vi "Target location.vi"(11 "Display map":dbl[][](array[numeric])) -> (2 "target location":dbl[](array[numeric]))   [LabVIEW 2015]
panel:
  in  "Priority map":dbl[][](array[numeric])
  in  "robot location":dbl[](array[numeric])
  out "distances":dbl[](array[numeric])
  out "Indices":i32[][](array[numeric])
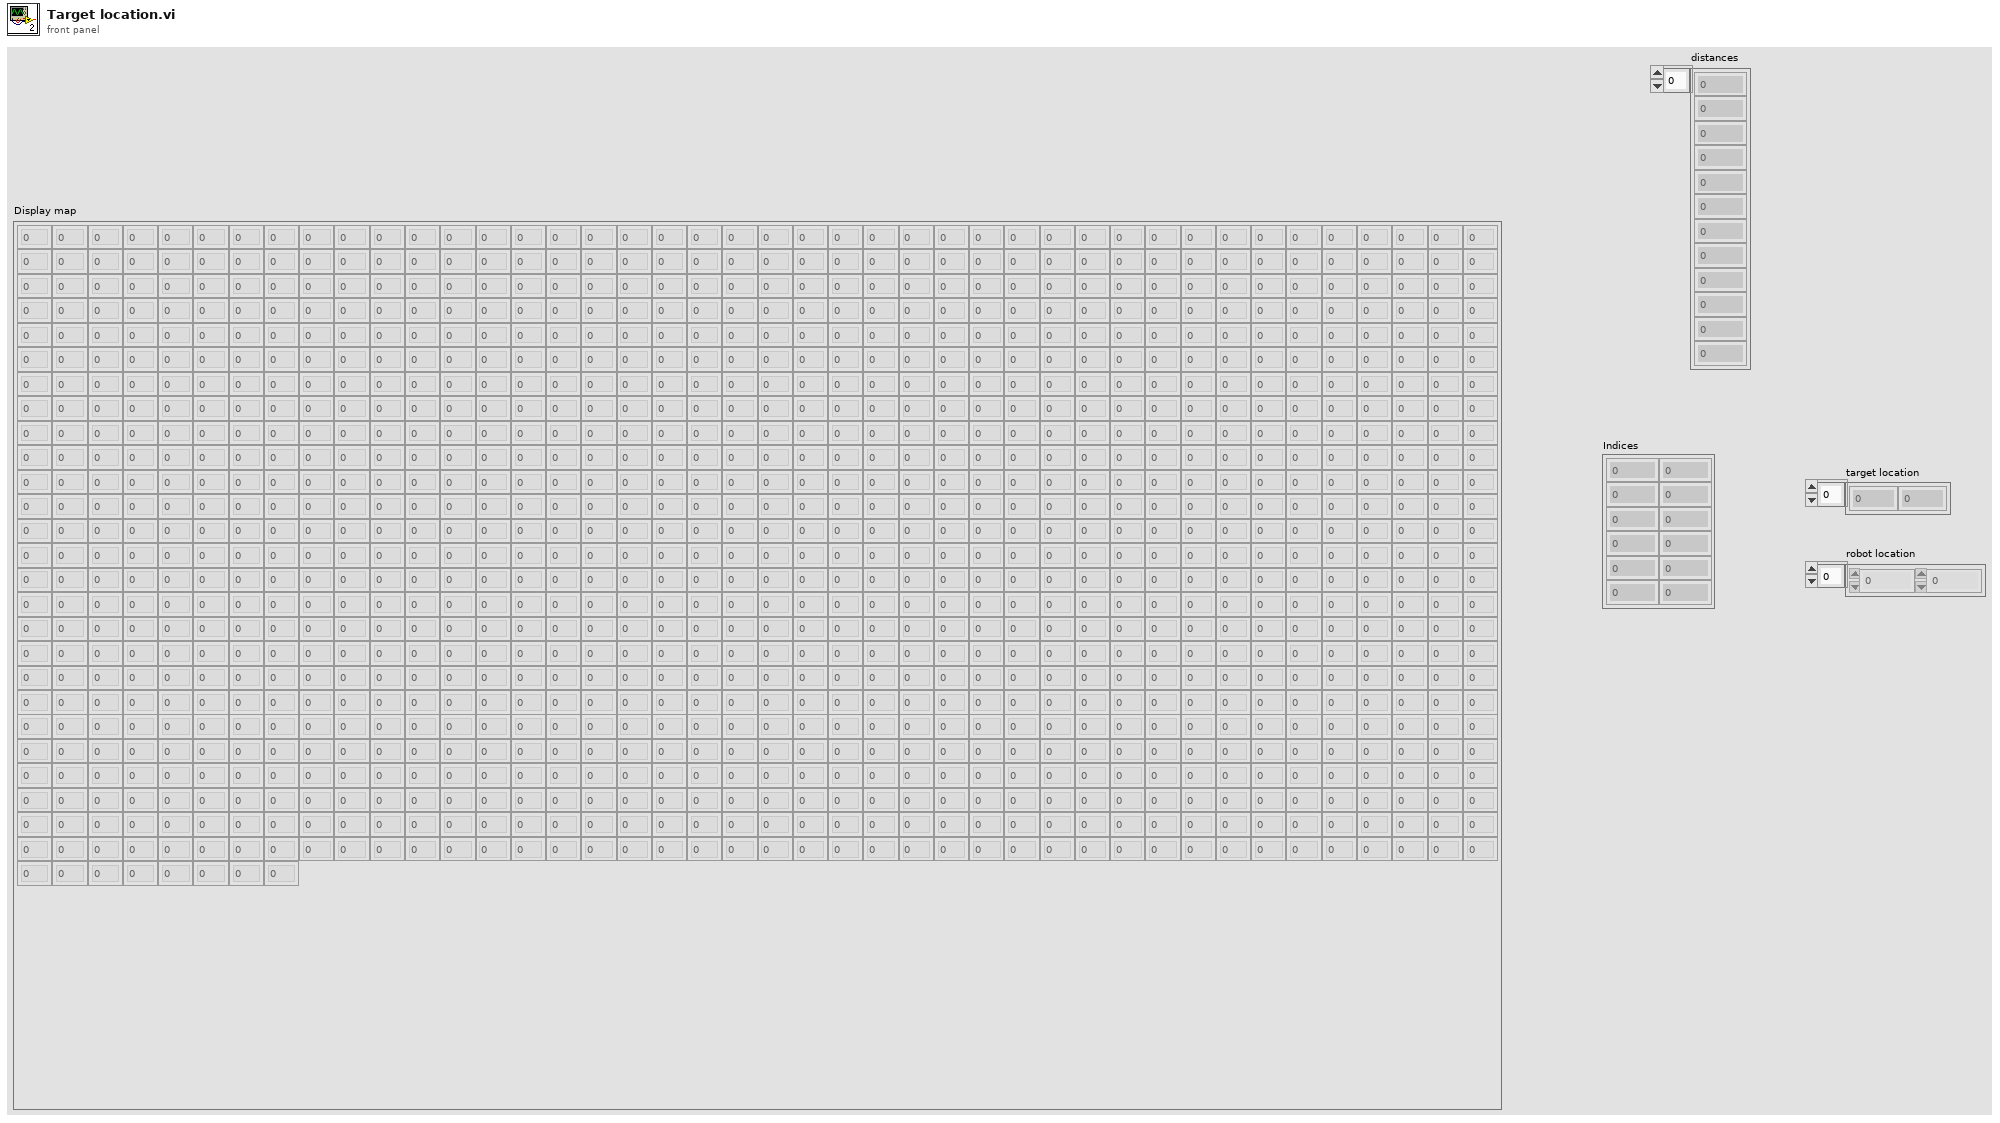
[diagram p1: front panel]
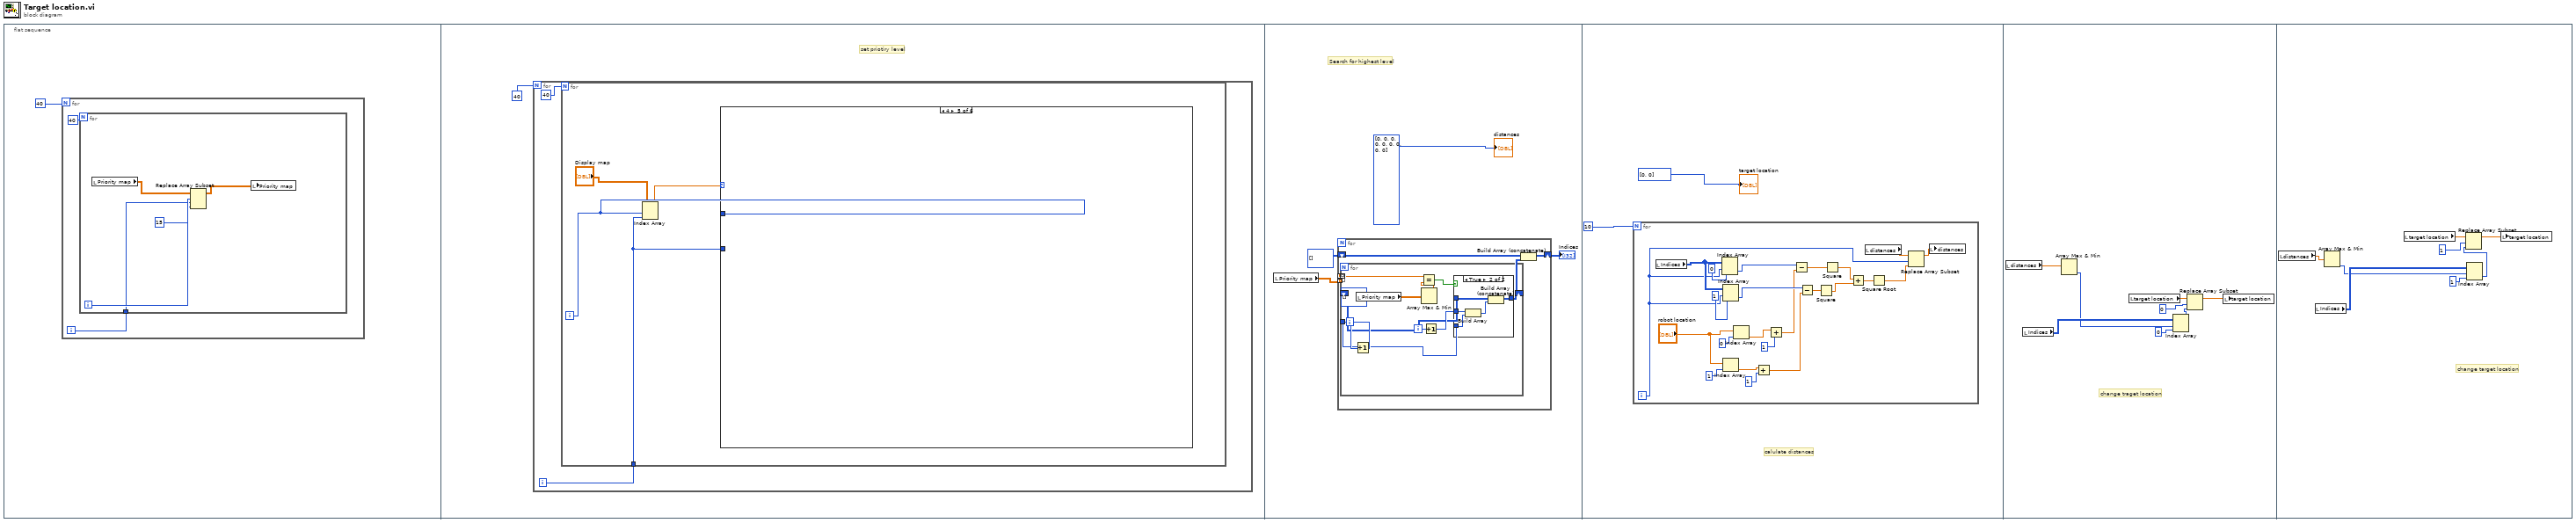
[diagram p0: block diagram]
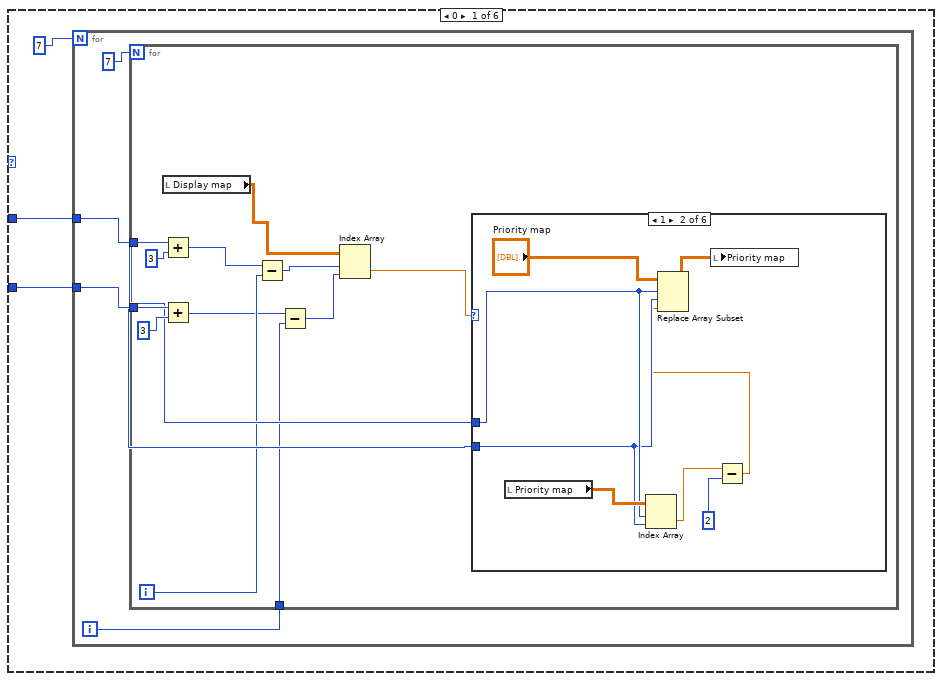
[diagram p2: hidden frame]
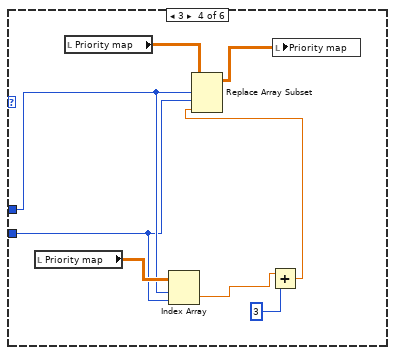
[diagram p5: hidden frame]
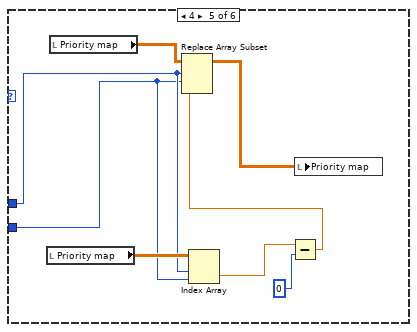
[diagram p6: hidden frame]
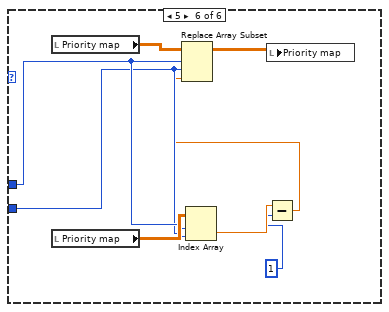
[diagram p7: hidden frame]
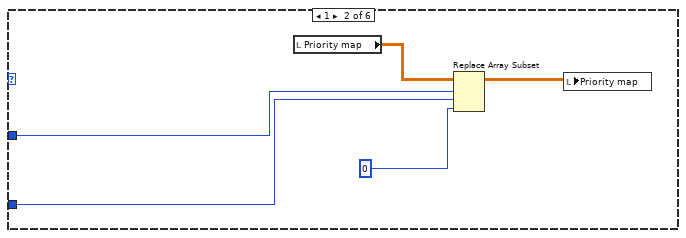
[diagram p8: hidden frame]
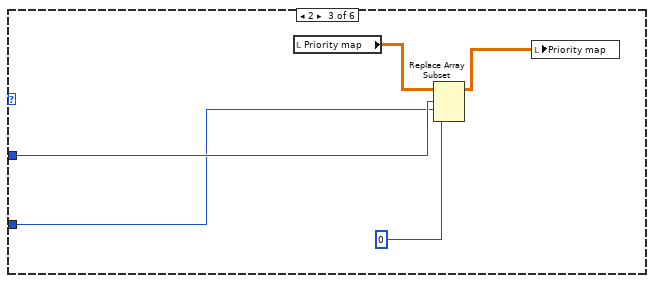
[diagram p9: hidden frame]
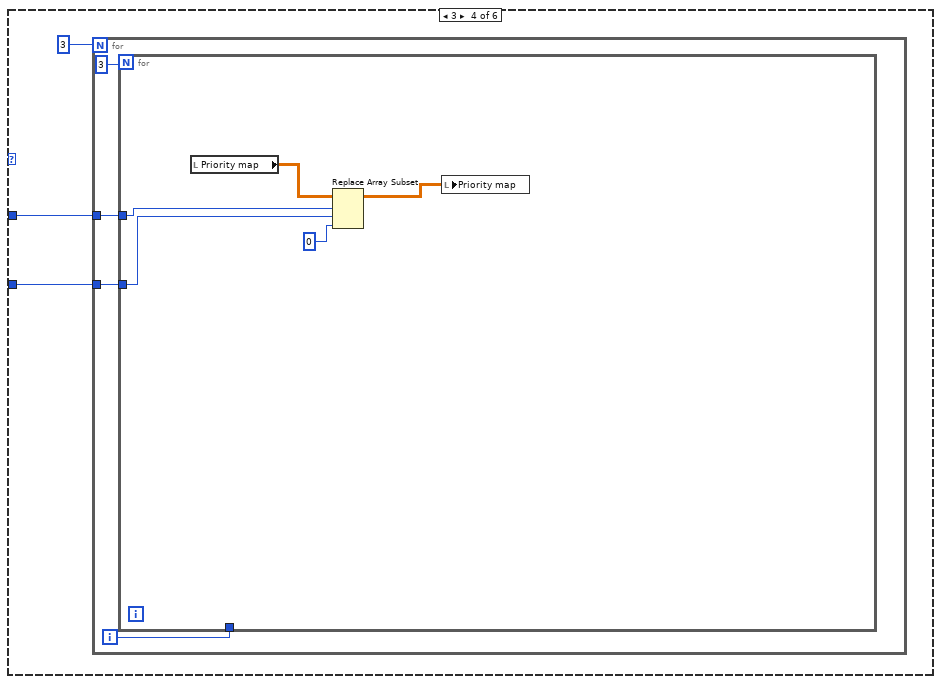
[diagram p10: hidden frame]
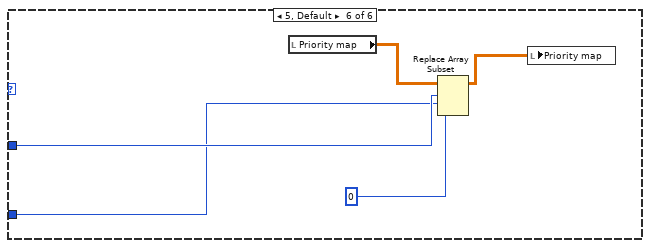
[diagram p11: hidden frame]
diagram:
  n1 = flat-sequence {
    frame #0 {
      n2 = for {
        N: 40 -> [_]
        i -> [w2]
        n3 = for {
          N: 40 -> [_]
          tunnel: w2 -> [w5]
          i -> [w6]
          n4 = local read "Priority map"() -> (w8:dbl[][])
          n5 = Replace Array Subset(array=w8, new element=15, index (row)=w6, index (col)=w5) -> (w7:dbl[][])
          n6 = local write "Priority map"(w7) -> ()
        }
      }
    }
    frame #1 {
      # "set priotiry level"
      n7 = for {
        N: 40 -> [_]
        i -> [w10]
        n8 = for {
          N: 40 -> [_]
          tunnel: w10 -> [w15]
          i -> [w14]
          n9 = Index Array(array="Display map", index (row)=w14, index (col)=w15) -> (element=w13:dbl)
          n10 = case shown="4" w13 {
            tunnel: w15 -> [w18 w68 w74 w79 _ w90]
            tunnel: w14 -> [w17 w67 w75 w78 _ w91]
            frame 0 {
              n11 = for {
                N: 7 -> [_]
                tunnel: w18 -> [w22]
                tunnel: w17 -> [w21]
                i -> [w19]
                n12 = for {
                  N: 7 -> [_]
                  tunnel: w22 -> [w31]
                  tunnel: w21 -> [w30]
                  tunnel: w19 -> [w26]
                  i -> [w28]
                  n13 = local read "Display map"() -> (w34:dbl[][])
                  n14 = Add(x=w30, y=3) -> (x+y=w29:i32)
                  n15 = Add(x=w31, y=3) -> (x+y=w27:i32)
                  n16 = Subtract(x=w29, y=w28) -> (x-y=w24:i32)
                  n17 = Subtract(x=w27, y=w26) -> (x-y=w25:i32)
                  n18 = Index Array(array=w34, index (row)=w24, index (col)=w25) -> (element=w23:dbl)
                  n19 = case shown="1" w23 {
                    tunnel: w31 -> [_ w39 _ w47 w55 w62]
                    tunnel: w30 -> [_ w40 _ w48 w56 w63]
                    frame 0, Default {
                    }
                    frame 1 {
                      n20 = local read "Priority map"() -> (w42:dbl[][])
                      n21 = Index Array(array=w42, index (row)=w40, index (col)=w39) -> (element=w38:dbl)
                      n22 = Subtract(x=w38, y=2) -> (x-y=w36:dbl)
                      n23 = Replace Array Subset(array="Priority map", new element=w36, index (row)=w40, index (col)=w39) -> (w41:dbl[][])
                      n24 = local write "Priority map"(w41) -> ()
                    }
                    frame 2 {
                    }
                    frame 3 {
                      n25 = local read "Priority map"() -> (w49:dbl[][])
                      n26 = local read "Priority map"() -> (w50:dbl[][])
                      n27 = Index Array(array=w49, index (row)=w48, index (col)=w47) -> (element=w46:dbl)
                      n28 = Add(x=w46, y=3) -> (x+y=w44:dbl)
                      n29 = Replace Array Subset(array=w50, new element=w44, index (row)=w48, index (col)=w47) -> (w45:dbl[][])
                      n30 = local write "Priority map"(w45) -> ()
                    }
                    frame 4 {
                      n31 = local read "Priority map"() -> (w57:dbl[][])
                      n32 = local read "Priority map"() -> (w58:dbl[][])
                      n33 = Index Array(array=w57, index (row)=w56, index (col)=w55) -> (element=w54:dbl)
                      n34 = Subtract(x=w54, y=0) -> (x-y=w53:dbl)
                      n35 = Replace Array Subset(array=w58, new element=w53, index (row)=w56, index (col)=w55) -> (w51:dbl[][])
                      n36 = local write "Priority map"(w51) -> ()
                    }
                    frame 5 {
                      n37 = local read "Priority map"() -> (w64:dbl[][])
                      n38 = local read "Priority map"() -> (w66:dbl[][])
                      n39 = Index Array(array=w66, index (row)=w63, index (col)=w62) -> (element=w61:dbl)
                      n40 = Subtract(x=w61, y=1) -> (x-y=w60:dbl)
                      n41 = Replace Array Subset(array=w64, new element=w60, index (row)=w63, index (col)=w62) -> (w65:dbl[][])
                      n42 = local write "Priority map"(w65) -> ()
                    }
                  }
                }
              }
            }
            frame 1 {
              n43 = local read "Priority map"() -> (w71:dbl[][])
              n44 = Replace Array Subset(array=w71, new element=0, index (row)=w67, index (col)=w68) -> (w70:dbl[][])
              n45 = local write "Priority map"(w70) -> ()
            }
            frame 2 {
              n46 = local read "Priority map"() -> (w76:dbl[][])
              n47 = Replace Array Subset(array=w76, new element=0, index (row)=w75, index (col)=w74) -> (w73:dbl[][])
              n48 = local write "Priority map"(w73) -> ()
            }
            frame 3 {
              n49 = for {
                N: 3 -> [_]
                tunnel: w79 -> [w83]
                tunnel: w78 -> [w82]
                i -> [w80]
                n50 = for {
                  N: 3 -> [_]
                  tunnel: w83 -> [w84]
                  tunnel: w82 -> [w85]
                  tunnel: w80 -> [_]
                  n51 = local read "Priority map"() -> (w88:dbl[][])
                  n52 = Replace Array Subset(array=w88, new element=0, index (row)=w85, index (col)=w84) -> (w87:dbl[][])
                  n53 = local write "Priority map"(w87) -> ()
                }
              }
            }
            frame 4 {
            }
            frame 5, Default {
              n54 = local read "Priority map"() -> (w93:dbl[][])
              n55 = Replace Array Subset(array=w93, new element=0, index (row)=w91, index (col)=w90) -> (w92:dbl[][])
              n56 = local write "Priority map"(w92) -> ()
            }
          }
        }
      }
    }
    frame #2 {
      # "Search for highest level"
      n57 = local read "Priority map"() -> (w96:dbl[][])
      n58 = for {
        tunnel: [w98] -> _ mode=indexing
        shift-right: [w102] -> w94
        shift-left: i32[][] [] -> [w100]
        tunnel: w96 -> [w98] mode=indexing
        i -> [w104]
        n59 = Increment(x=w104) -> (x+1=w103:i32)
        n60 = for {
          tunnel: w98 -> [w113] mode=indexing
          tunnel: w103 -> [w109]
          shift-right: [w108] -> w101
          shift-left: i32[][] [] -> [w107]
          i -> [w111]
          n61 = local read "Priority map"() -> (w106:dbl[][])
          n62 = Array Max & Min(array=w106) -> (max value=w105:dbl)  [unwired: 3 out]
          n63 = Equal?(x=w113, y=w105) -> (x = y?=w112:bool)
          n64 = Increment(x=w111) -> (x+1=w110:i32)
          n65 = case shown="True" w112 {
            tunnel: w110 -> [_ w119]
            tunnel: w109 -> [_ w118]
            tunnel: [w114 w116] -> w108
            tunnel: w107 -> [w114 w115]
            frame False {
            }
            frame True {
              n66 = Build Array(w119, w118) -> (w117:i32[])
              n67 = Build Array (concatenate)(w115, w117) -> (w116:i32[][])
            }
          }
        }
        n68 = Build Array (concatenate)(w100, w101) -> (w102:i32[][])
      }
      "Indices" <- w94
      "distances" <- i32[] [0, 0, 0, 0, 0, 0, 0, 0, 0]
    }
    frame #3 {
      # "calulate distances"
      n69 = for {
        N: 10 -> [_]
        i -> [w122]
        n70 = local read "Indices"() -> (w144:i32[][])
        n71 = Index Array(array=w144, index (row)=w122, index (col)=0) -> (element=w136:i32)
        n72 = Index Array(array=w144, index (row)=w122, index (col)=1) -> (element=w135:i32)
        n73 = Index Array(array="robot location", index=1) -> (element=w138:dbl)
        n74 = Index Array(array="robot location", index=0) -> (element=w140:dbl)
        n75 = Add(x=w138, y=1) -> (x+y=w133:dbl)
        n76 = Add(x=w140, y=1) -> (x+y=w134:dbl)
        n77 = Subtract(x=w136, y=w134) -> (x-y=w132:dbl)
        n78 = Subtract(x=w135, y=w133) -> (x-y=w125:dbl)
        n79 = Square(x=w125) -> (x^2=w131:dbl)
        n80 = Square(x=w132) -> (x^2=w130:dbl)
        n81 = Add(x=w130, y=w131) -> (x+y=w129:dbl)
        n82 = local read "distances"() -> (w128:dbl[])
        n83 = Square Root(x=w129) -> (sqrt(x)=w126:dbl)
        n84 = Replace Array Subset(array=w128, new element=w126, index=w122) -> (w127:dbl[])
        n85 = local write "distances"(w127) -> ()
      }
      "target location" <- i32[] [0, 0]
    }
    frame #4 {
      # "change traget location"
      n86 = local read "distances"() -> (w145:dbl[])
      n87 = local read "Indices"() -> (w152:i32[][])
      n88 = Array Max & Min(array=w145) -> (min index (indices)=w150:i32)  [unwired: 3 out]
      n89 = local read "target location"() -> (w148:dbl[])
      n90 = Index Array(array=w152, index (row)=w150, index (col)=0) -> (element=w147:i32)
      n91 = Replace Array Subset(array=w148, new element=w147, index=0) -> (w146:dbl[])
      n92 = local write "target location"(w146) -> ()
    }
    frame #5 {
      # "change target location"
      n93 = local read "distances"() -> (w154:dbl[])
      n94 = local read "Indices"() -> (w155:i32[][])
      n95 = Array Max & Min(array=w154) -> (min index (indices)=w153:i32)  [unwired: 3 out]
      n96 = local read "target location"() -> (w158:dbl[])
      n97 = Index Array(array=w155, index (row)=w153, index (col)=1) -> (element=w159:i32)
      n98 = Replace Array Subset(array=w158, new element=w159, index=1) -> (w160:dbl[])
      n99 = local write "target location"(w160) -> ()
    }
  }
